vi "U-I-State.vi"(8 "error in (no error)":errorcluster, 11 "CS++DCPwrChannelData in":refnum<class "CS++DCPwrChannelData.lvclass">) -> (0 "error out":errorcluster, 2 "Actual Measurements":T1(array[cluster]), 3 "CS++DCPwrChannelData out":refnum<class "CS++DCPwrChannelData.lvclass">)   [LabVIEW 2015, in "CS++DCPwrGui.lvlib" / "CS++DCPwrChannelData.lvclass"]
uses:
  CS++DCPwrChannelData.lvclass
  CS++DCPwrChannelData.lvclass/CS++DCPwrChannelData.ctl
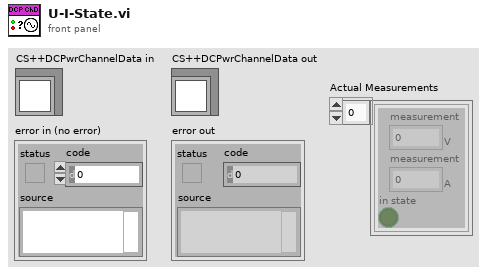
[diagram p1: front panel]
types:
  T1 = cluster{"measurement":dbl[unit], "measurement":dbl[unit], "in state":bool}[]
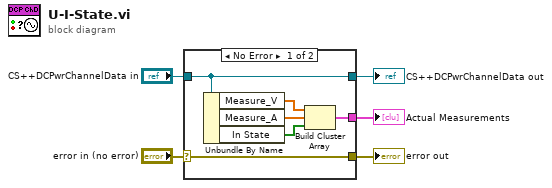
[diagram p0: block diagram]
diagram:
  n1 = case shown="No Error" "error in (no error)" {
    selector: "error in (no error)" -> [w11 w13]
    tunnel: [w11 w13] -> w4
    tunnel: [w10 w12] -> w2
    tunnel: "CS++DCPwrChannelData in" -> [w10 w12]
    tunnel: [w6 _] -> w1
    frame No Error {
      n2 = Unbundle By Name(w10) -> ("Measure_V"=w9:dbl[unit][], "Measure_A"=w8:dbl[unit][], "In State"=w7:bool[])
      n3 = Build Cluster Array(w9, w8, w7) -> (w6:T1)
    }
    frame Error {
    }
  }
  "error out" <- w4
  "CS++DCPwrChannelData out" <- w2
  "Actual Measurements" <- w1
